vi "Ambient Light Bricklet Sandbox.vi"() -> ()   [LabVIEW 2011]
uses:
  Classes/Ambient Light Bricklet/Properties/Read CB illuminance.vi
  Classes/Ambient Light Bricklet/Ambient Light Bricklet.lvclass
  Classes/IP Connection/IP Connection.lvclass
panel:
  out "Waveform Chart":dbl(graph)
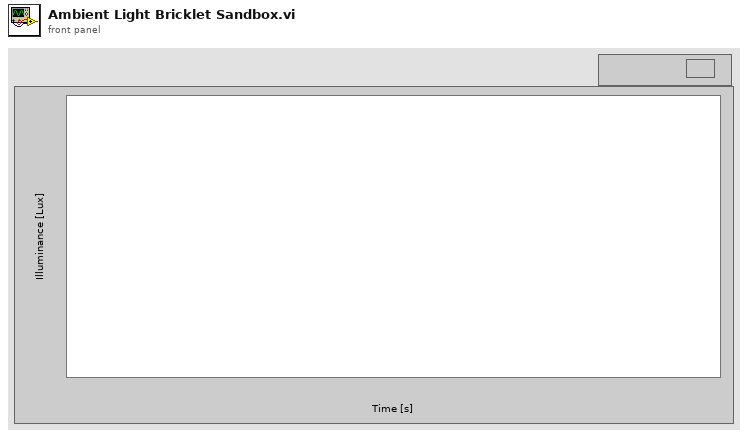
[diagram p1: front panel]
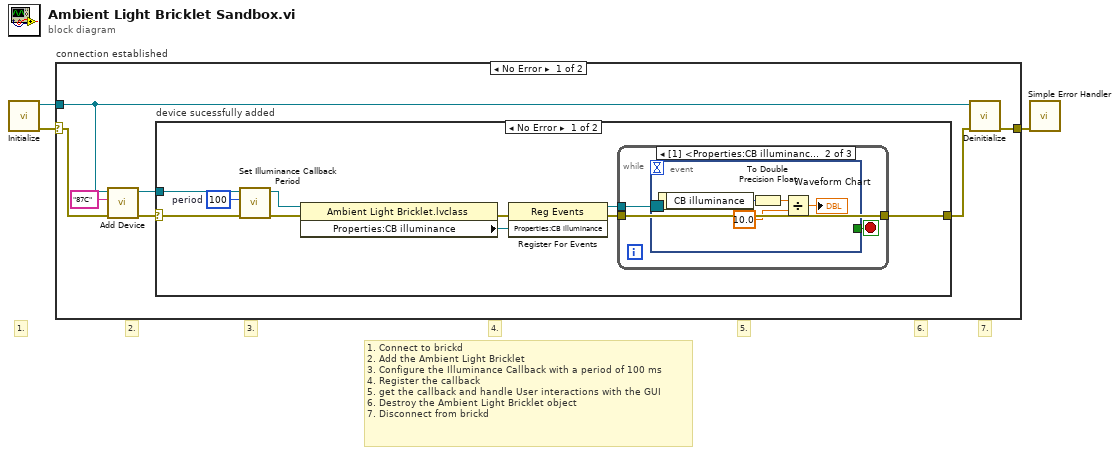
[diagram p0: block diagram]
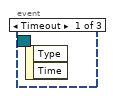
[diagram p2: hidden frame]
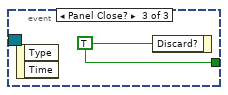
[diagram p3: hidden frame]
diagram:
  # "7."
  # "1. Connect to brickd\n2. Add the Ambient Light Bricklet\n3. Configure the Illuminance Callback with a period of 100 ms\n4. Register the callback\n5. get the callback and handle User interactions with the GUI\n6. Destroy the Ambient Light Bricklet object \n7. Disconnect from brickd"
  # "6."
  # "5."
  # "4."
  # "3."
  # "2."
  # "1."
  n1 = call "Initialize.vi"() -> ("error out"=w1:errorcluster, "IP Connection out"=w3:refnum<class "IP Connection.lvclass">)  [unwired: 10 in]
  n2 = case "connection established" shown="No Error" w1 {
    selector: w1 -> [w5 w30]
    tunnel: w3 -> [w10 _]
    tunnel: [w9 w30] -> w2
    frame No Error {
      n3 = call "Add Device.vi"("Error In"=w5, "Device UID"="87C", "IP Connection"=w10) -> ("Error Out"=w4:errorcluster, "Ambient Light Bricklet"=w6:refnum<class "Ambient Light Bricklet.lvclass">)  [unwired: 7 in]
      n4 = case "device sucessfully added" shown="No Error" w4 {
        selector: w4 -> [w12 w29]
        tunnel: [w11 w29] -> w7
        tunnel: w6 -> [w16 _]
        frame No Error {
          w15 = u32 100  # period
          n5 = call "Set Illuminance Callback Period.vi"("error in (no error)"=w12, "period (0: off)"=w15, "Ambient Light Bricklet in"=w16) -> ("error out"=w14:errorcluster, "Ambient Light Bricklet out"=w13:refnum<class "Ambient Light Bricklet.lvclass">)  [unwired: 7 in]
          n6 = property class="Ambient Light Bricklet.lvclass"(reference=w13, error in=w14) -> (error out=w20:errorcluster, "Properties:CB illuminance"=w19:refnum<user-event>)  [unwired: 1 out]
          n7 = register-events(error in=w20, w19) -> (reference out=w17:refnum<event-registration>, error out=w18:errorcluster)  [unwired: 1 in]
          n8 = while {
            tunnel: w18 -> [w21]
            tunnel: w17 -> [w22]
            tunnel: [w21] -> w11
            stop <- w23 stop-if-true
            n9 = event shown="[1] <Properties:CB illuminance>: User Event" {
              selector: w22 -> [_ _ _]
              dyn-events: _ -> [_ _ _]
              timeout: _ -> [_ _ _]
              tunnel: [_ _ w28] -> w23
              event Timeout {
                n10 = event-data() -> ()  [unwired: 1 in, 2 out]
              }
              event User Event {
                n11 = event-data() -> ("CB illuminance"=w27:u16)  [unwired: 1 in]
                n12 = To Double Precision Float(number=w27) -> (double precision float=w25:dbl)
                n13 = Divide(x=w25, y=10.0) -> (x/y=→"Waveform Chart":dbl)
              }
              event Panel Close? {
                w28 = TRUE ("Discard?")
                n14 = event-data() -> ()  [unwired: 1 in, 2 out]
                n15 = event-data("Discard?"=w28) -> ()  [unwired: 1 in, 1 out]
              }
            }
          }
        }
        frame Error {
        }
      }
      n16 = call "Deinitialize.vi"("error in (no error)"=w7, "IP Connection in"=w10) -> ("error out"=w9:errorcluster)  [unwired: 9 in]
    }
    frame Error {
    }
  }
  n17 = call <vilib>:"Simple Error Handler.vi"("error in (no error)"=w2) -> ()  [unwired: 4 in, 5 out]
